vi "Core.vi"(8 "error in (no error)":errorcluster, 10 "Actor in":refnum<class "Actor.lvclass">, 11 "Multi Instrument Msg in":refnum<class "Multi Instrument Msg.lvclass">) -> (0 "error out":errorcluster, 1 "Data":refnum<class "Data.lvclass">, 2 "Actor out":refnum<class "Actor.lvclass">, 3 "Multi Instrument Msg out":refnum<class "Multi Instrument Msg.lvclass">)   [LabVIEW 2020, in "Instrument Handler.lvlib" / "Multi Instrument Msg.lvclass"]
doc: "Core of the Reponse Msg. Put the active code here.\n\nThis implementation extract the Instrument from the Instrument Owner or Handler and calls Instrument Do Core, where the actual instrument interaction takes place, or calls the Owners indrectly from Multi Instrument Do Core."
uses:
  Multi Instrument Msg.lvclass
  C:/Current projects/WS/Framework/Framework/Actors/Instrument Handler/Messages/Instrument Msg/Instrument Msg.lvclass
  PPL/HDH.Data.Generic.lvlibp/Data.lvclass
  PPL/HDH.Actor Framework.Core.Actor.lvlibp/1abvi3w/vi.lib/ActorFramework/Actor/Actor.lvclass
  Multi Instrument Handler/Multi Instrument Handler.lvclass
  Instrument Msg/Instrument Msg.lvclass
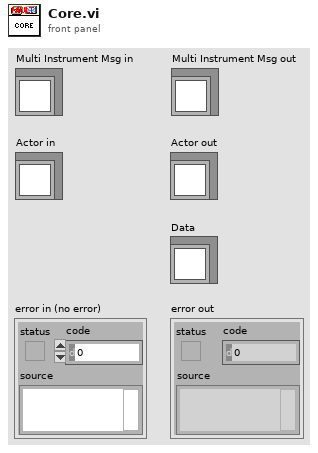
[diagram p1: front panel]
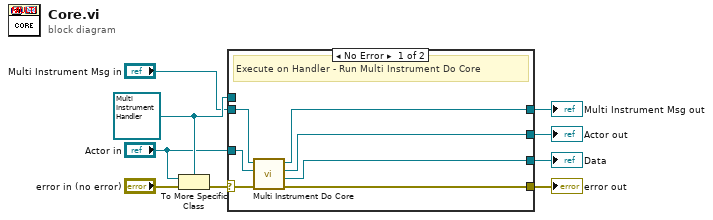
[diagram p0: block diagram]
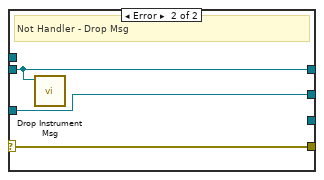
[diagram p2: hidden frame]
diagram:
  w8 = refnum<class "Multi Instrument Handler.lvclass"> refnum ("Instrument Handler.lvlib:Multi Instrument Handler.lvclass")
  n1 = To More Specific Class(target class=w8, reference="Actor in", error in="error in (no error)") -> (error out=w9:errorcluster)  [unwired: 1 out]
  n2 = case shown="No Error" w9 {
    selector: w9 -> [w10 w19]
    tunnel: [w13 w19] -> w1
    tunnel: "Multi Instrument Msg in" -> [w16 w18]
    tunnel: [w15 w18] -> w4
    tunnel: [w14 w17] -> w3
    tunnel: "Actor in" -> [w11 w17]
    tunnel: w8 -> [_ _]
    tunnel: [w12 _] -> w2
    frame No Error {
      # "Execute on Handler - Run Multi Instrument Do Core"
      n3 = call-dynamic "Multi Instrument Do Core.vi"("error in (no error)"=w10, "Actor in"=w11, "Instrument Msg in"=w16) -> ("error out"=w13:errorcluster, "Data"=w12:refnum<class "Data.lvclass">, "Actor out"=w14:refnum<class "Actor.lvclass">, "Instrument Msg out"=w15:refnum<class "Multi Instrument Msg.lvclass">)  [unwired: 5 in]
    }
    frame Error {
      # "Not Handler - Drop Msg"
      n4 = call "Drop Instrument Msg.vi"("Instrument Msg in"=w18) -> ()  [unwired: 11 in]
    }
  }
  "error out" <- w1
  "Actor out" <- w3
  "Data" <- w2
  "Multi Instrument Msg out" <- w4
